vi "Retrieve Process from App.vi"(8 "error in (no error)":errorcluster, 10 "String":string, 11 "Application In":refnum<class "Application.lvclass">) -> (0 "error out":errorcluster, 2 "Process":refnum<class "Process.lvclass">, 3 "Application Out":refnum<class "Application.lvclass">)   [LabVIEW 2020, in "Application.lvclass"]
uses:
  Application.lvclass
  C:/git/astemes-triarc-framework/source/Framework/Process/Process.lvclass
  Process/Process.lvclass
  C:/git/astemes-triarc-framework/source/Framework/Logging/Logging.lvclass
  Application.lvclass/Application.ctl
  Process/Process.lvclass/Process.ctl
  Process/Protected/Messaging/Async Request Message.vi
  Process/Private/SubVIs/Handle Debug Data.vi
  Logging/Log Debug.vi
  <vilib>/AdvancedString/1D String Array to Delimited String.vi
  <vilib>/Utility/High Resolution Relative Seconds.vi
  Synchronous Request Callback/Synchronous Request Callback.lvclass
  C:/git/astemes-triarc-framework/source/Framework/Callback/Callback.lvclass
  <vilib>/Utility/error.llb/Error Cluster From Error Code.vi
  Process/Public/Lifecycle/Get Lifecycle State.vi
  Synchronous Request Callback/Create.vi
  Process/Public/Read Name.vi
  Process/Private/SubVIs/Wait for Response Message.vi
  <vilib>/ErrorRing/Error Ring.xnode
  Callback/Callback.lvclass
  Logging/Logging.lvclass
  C:/git/astemes-triarc-framework/source/Framework/Base/Base.lvclass
  C:/git/astemes-triarc-framework/source/Framework/Error Handler Interface/Error Handler Interface.lvclass
  C:/git/astemes-triarc-framework/source/Framework/Application/Application.lvclass
  C:/git/astemes-triarc-framework/source/Framework/Async Handler/Async Handler.lvclass
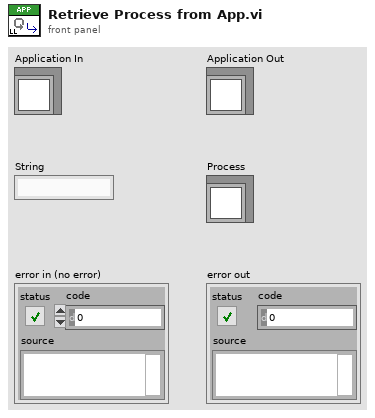
[diagram p1: front panel]
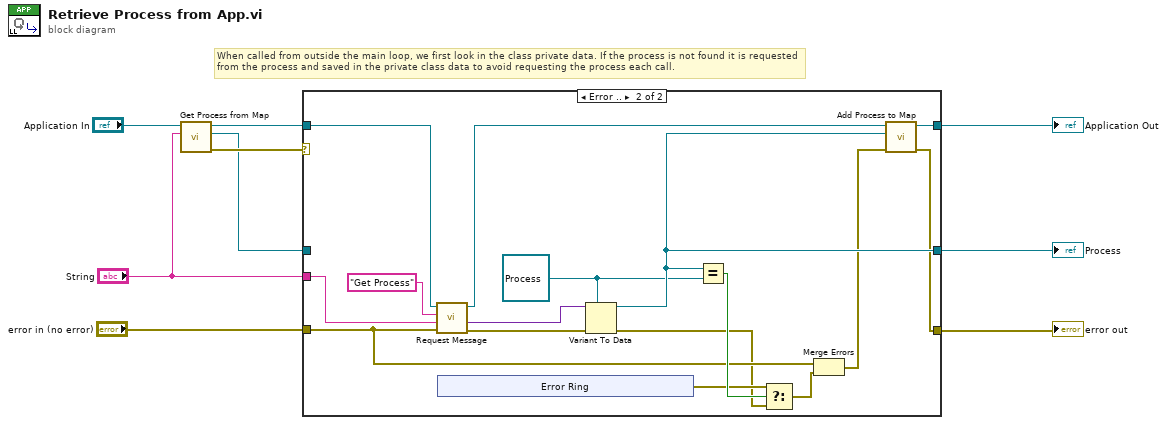
[diagram p0: block diagram]
diagram:
  # "When called from outside the main loop, we first look in the class private data. If the process is not found it is requested from the process and saved in the private class data to avoid requesting the process each call."
  n1 = call "Get Process from Map.vi"("Process Name"="String", "Application In"="Application In") -> ("error out"=w3:errorcluster, "Process"=w2:refnum<class "Process.lvclass">, "Application Out"=w4:refnum<class "Application.lvclass">)  [unwired: 7 in]
  n2 = case shown="Error .." w3 {
    tunnel: [w12 w13] -> w8
    tunnel: [w10 w21] -> w6
    tunnel: "error in (no error)" -> [w12 w16]
    tunnel: w4 -> [w11 w25]
    tunnel: "String" -> [_ w24]
    tunnel: w2 -> [w10 _]
    tunnel: [w11 w22] -> w7
    frame No Error {
      # "Or we have not started process"
      # "Or we are in process loop"
      # "Process has been requested before and is found in current object"
    }
    frame Error {
      w20 = refnum<class "Process.lvclass"> refnum ("Rig Process")
      n3 = call "Request Message.vi"("error in (no error)"=w16, "Request Message Data"=w24, "Request Message"="Get Process", "Process In"=w25) -> ("error out"=w28:errorcluster, "Response Message Data"=w26:variant, "Process Out"=w23:refnum<class "Application.lvclass">)  [unwired: 3 in, 2 out]
      n4 = xnode "Error Ring"() -> ("error out"=w18:errorcluster)
      n5 = Variant To Data(error in=w28, type=w20, Variant=w26) -> (data=w21:refnum<class "Process.lvclass">, error out=w15:errorcluster)
      n6 = Equal?(x=w21, y=w20) -> (x = y?=w19:bool)
      n7 = Select(t=w18, s=w19, f=w15) -> (s? t:f=w17:errorcluster)
      n8 = Merge Errors(w16, w17) -> (w14:errorcluster)
      n9 = call "Add Process to Map.vi"("error in (no error)"=w14, "Process Out"=w21, "Application In"=w23) -> ("error out"=w13:errorcluster, "Application Out"=w22:refnum<class "Application.lvclass">)  [unwired: 7 in]
    }
  }
  "error out" <- w8
  "Application Out" <- w7
  "Process" <- w6
